vi "Update from GIT.vi"(1 "Branch name":string, 2 "Update GIT":bool) -> ()   [LabVIEW 2026, in "TALOS.lvlib" / "Guardian.lvlib" / "Guardian.lvclass"]
uses:
  Guardian.lvclass
  <vilib>/Utility/LVLibp/NI_PackedLibraryUtility.lvlib
  TALOS.lvlib
panel:
  out "error out":errorcluster
  # "1) Close LabView (this operation will ignores the state of the files,\nmeaning all unsaved changes will most likely be lost).\n2) If the flag is true update code in the git repository on the current branch.\nIt does git reset --hard & git pull\n3) Start guardian with the Startup.bat file"
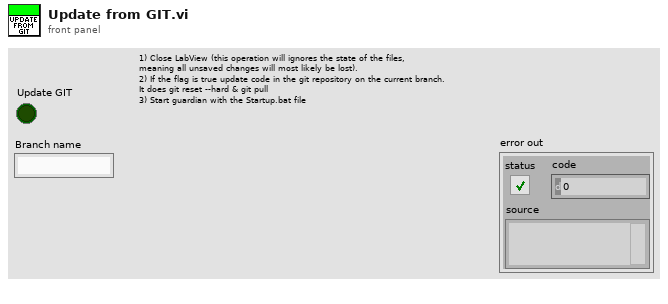
[diagram p1: front panel]
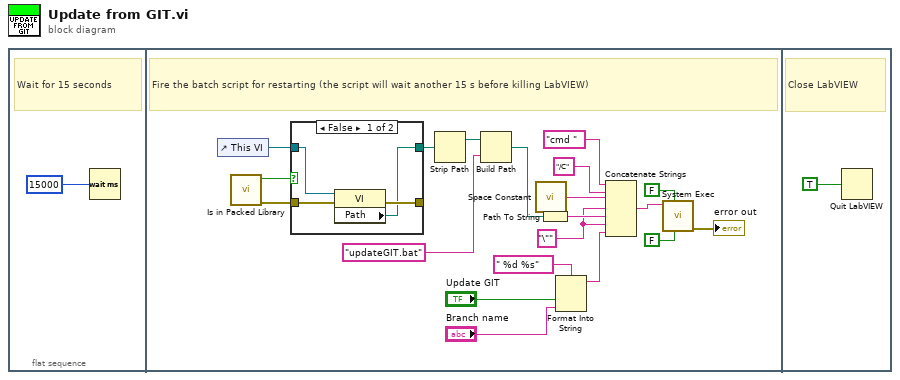
[diagram p0: block diagram]
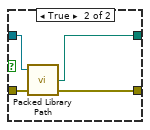
[diagram p2: hidden frame]
diagram:
  n1 = flat-sequence {
    frame #0 {
      # "Wait for 15 seconds"
      n2 = Wait (ms)(milliseconds to wait=u32 15000) -> ()  [unwired: 1 out]
    }
    frame #1 {
      w8 = "\"" ("string")
      # "Fire the batch script for restarting (the script will wait another 15 s before killing LabVIEW)"
      n3 = control-ref of="This VI"() -> (w14:refnum<vi>)
      n4 = call "Is in Packed Library.vi"() -> ("error out"=w13:errorcluster, "Is In Packed Library"=w4:bool)  [unwired: 10 in]
      n5 = case shown="False" w4 {
        tunnel: w13 -> [w24 w29]
        tunnel: [w25 w27] -> _
        tunnel: [w22 w28] -> w15
        tunnel: w14 -> [w23 w26]
        frame False {
          n6 = property class="VI"(reference=w23, error in=w24) -> (error out=w25:errorcluster, "Path"=w22:path)  [unwired: 1 out]
        }
        frame True {
          n7 = call <vilib>:"Packed Library Path.vi"("error in (no error)"=w29, "vi reference"=w26) -> ("error out"=w27:errorcluster, "packed library path"=w28:path)  [unwired: 1 in, 1 out]
        }
      }
      n8 = Strip Path(path=w15) -> (stripped path=w12:path)  [unwired: 1 out]
      n9 = Build Path(base path=w12, name or relative path="updateGIT.bat" ("string")) -> (appended path=w10:path)
      n10 = call <vilib>:"Space Constant.vi"() -> ("String"=w7:string)
      n11 = Path To String(path=w10) -> (string=w9:string)
      n12 = Format Into String(format string=" %d %s", "Update GIT", "Branch name") -> (resulting string=w3:string)  [unwired: 2 in, 1 out]
      n13 = Concatenate Strings("cmd " ("string"), "/C" ("string"), w7, w8, w9, w8, w3) -> (w19:string)
      n14 = call <vilib>:"System Exec.vi"("run minimized? (F)"=FALSE, "wait until completion? (T)"=FALSE, "command line"=w19) -> ("error out"=→"error out":errorcluster)  [unwired: 5 in, 3 out]
    }
    frame #2 {
      # "Close LabVIEW"
      n15 = Quit LabVIEW(quit? (T)=TRUE) -> ()
    }
  }
